vi "p1.vi"() -> ()   [LabVIEW 2023, in "d16.lvlib"]
uses:
  d16.lvlib
  AOC/AOC.lvlib
panel:
  in  "Example":string=".|...\\....\n|.-.\\.....\n.....|-...\n........|.\n..........\n.........\\\n..../.\\\\..\n.-.-/..|..\n.|....-|.\\\n..//.|...."
  in  "Example":bool=TRUE
  out "Answer":u64=15
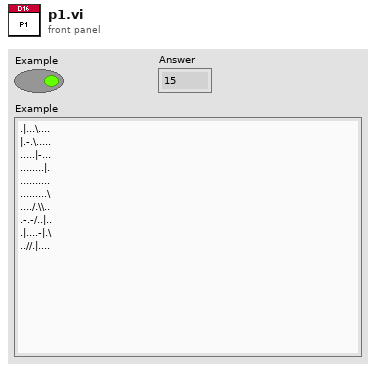
[diagram p1: front panel]
types:
  T1 = cluster{"position":cluster{"x":i32, "y":i32}, "direction":string}
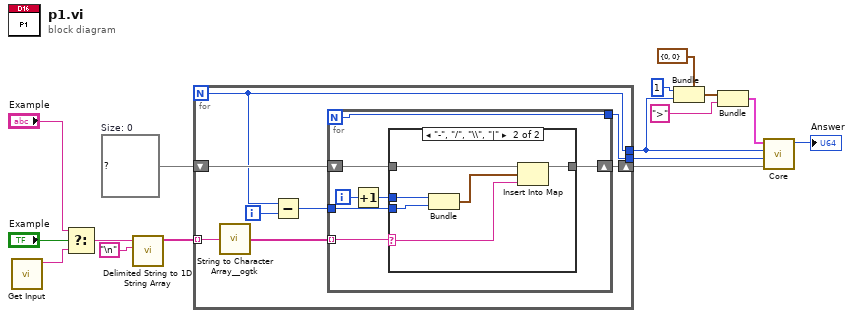
[diagram p0: block diagram]
diagram:
  w10 = map{cluster{i32, i32}, string} {}  # Size: 0
  n1 = call "Get Input.vi"() -> ("Input"=w16:string)  [unwired: 11 in]
  n2 = Select(t="Example", s="Example", f=w16) -> (s? t:f=w15:string)
  n3 = call <vilib>:"Delimited String to 1D String Array.vi"("delimiter"="\n", "delimited string"=w15) -> ("string array"=w11:string[])  [unwired: 9 in]
  n4 = for {
    N -> [w17]
    tunnel: w11 -> [w24] mode=indexing
    shift-right: [w20] -> w2
    shift-left: w10 -> [w21]
    tunnel: [w17] -> w4
    tunnel: [w19] -> w3
    i -> [w22]
    n5 = call <userlib>:"String to Character Array__ogtk.vi"("Input String"=w24) -> ("Character Array"=w23:string[])
    n6 = Subtract(x=w17, y=w22) -> (x-y=w18:i32)
    n7 = for {
      N -> [w26]
      tunnel: w23 -> [w31] mode=indexing
      tunnel: w18 -> [w29]
      shift-right: [w27] -> w20
      shift-left: w21 -> [w28]
      tunnel: [w26] -> w19
      i -> [w30]
      n8 = Increment(x=w30) -> (x+1=w25:i32)
      n9 = case shown="\"-\", \"/\", \"\\\\\", \"|\"" w31 {
        selector: w31 -> [_ w36]
        tunnel: w25 -> [_ w38]
        tunnel: w29 -> [_ w37]
        tunnel: w28 -> [w32 w35]
        tunnel: [w32 w34] -> w27
        frame Default {
        }
        frame "-", "/", "\\", "|" {
          n10 = Bundle(w38, w37) -> (w33:cluster{i32, i32})  [unwired: 1 in]
          n11 = Insert Into Map(map in=w35, key=w33, value=w36) -> (map out=w34:map{cluster{i32, i32}, string})  [unwired: 2 out]
        }
      }
    }
  }
  n12 = Bundle(cluster=cluster{"x":i32, "y":i32} {"x"=0, "y"=0} ("position"), "x"=1, "y"=w4) -> (w7:cluster{"x":i32, "y":i32})
  n13 = Bundle("position"=w7, "direction"=">") -> (w5:T1)  [unwired: 1 in]
  n14 = call "Core.vi"("Mirrors& Splitters"=w2, "ySize"=w3, "xSize"=w4, "Initial Lazer"=w5) -> ("Number Energized"=→"Answer":i32)  [unwired: 7 in]
